vi "ni5660 Configure for Spectrum.vi"(0 "receiver info in":T1, 1 "advanced settings":T3={"window"=enum."7 Term B-Harris", "spectral lines"=-1, "RBW definition"=enum."3dB"}, 5 "center frequency (Hz)":dbl=100000000.0 format="%.2p", 7 "span (Hz)":dbl=20000000.0 format="%.2p", 9 "resolution bandwidth (Hz)":dbl=100000.0 format="%.2p", 11 "error in (no error)":errorcluster, 12 "reference level (dBm)":i32, 13 "auto attenuation":enum16{"DISABLE", "ENABLE"}(ring)=enum."ENABLE", 14 "attenuation (dB)":i32=20) -> (4 "receiver info out":T1, 8 "actual resolution bandwidth (Hz)":dbl, 10 "correction factor":T2[](array[typedef]) {"spectrum correction"."correction factors" format="%.2f"; "spectrum correction"."df" format="%.2f"; "spectrum correction"."f0" format="%.2f"}, 15 "error out":errorcluster)   [LabVIEW 2011]
doc: "This VI configures the RF Signal Analyzer hardware to acquire a frequency-domain spectrum with spectral settings you specify.<B> Center frequency</B>, <B>span</B>, and <B>resolution bandwidth</B> parameter settings define the spectrum. You can also specify window type, number of spectral lines, and resolution bandwidth (RBW) definition. \n\nThis VI configures the reference level and attenuation settings used by the RF downconverter module, and the horizontal settings and acquisition type used by the IF digitizer module. It returns a <B>correction factor</B> array. Wire this output to the <B>correction factor</B> input parameter of the ni5660 Read Averaged Power Spectrum VI or ni5660 Read FFT Spectrum VI."
uses:
  <vilib>/addons/Spectral Measurements Toolset/LVSupport/SMT niScope Utilities/smt_correction.ctl
  <vilib>/addons/Modulation/niScope/controls/mod_Modulation Settings.ctl
  <vilib>/addons/Spectral Measurements Toolset/LVSupport/SMT niScope Utilities/SMT niScope Dependent/SMT Config niScope for Spectrum(auto).vi
  <instrlib>/NITUNER/niTuner Get Cal.vi
  <instrlib>/NITUNER/niTuner Set Freq.vi
  <vilib>/Analysis/1siggen.llb/Ramp Pattern by Samples.vi
  <vilib>/addons/Spectral Measurements Toolset/LVSupport/SMT niScope Utilities/SMT Calculate Correction(Zoom FFT).vi
  <vilib>/addons/Spectral Measurements Toolset/LVSupport/SMT niScope Utilities/SMT RFSA Dependent/SMT Configure RFSA for Spectrum(auto).vi
  <vilib>/Analysis/NI_AALBase.lvlib
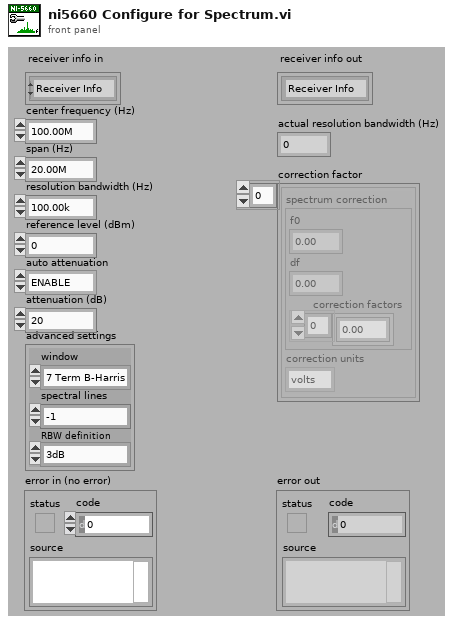
[diagram p1: front panel]
types:
  T1 = typedef "mod_Modulation Settings.ctl" = cluster{enum16{"Receiver Info"}, variant}
  T2 = typedef "smt_correction.ctl" = cluster{"spectrum correction":cluster{"f0":dbl, "df":dbl, "correction factors":dbl[]}, "correction units":enum16{"volts", "watts", "dB"}}
  T3 = cluster{"window":enum16{"None ", "Hanning", "Hamming", "Blackman-Harris", "Exact Blackman", "Blackman", "Flat Top", "4 Term B-Harris ", "7 Term B-Harris", "Low Sidelobe"}, "spectral lines":i32, "RBW definition":enum16{"3dB", "6dB", "ENBW", "bin width"}}
  T4 = cluster{"window":enum16{"None ", "Hanning", "Hamming", "Blackman-Harris", "Exact Blackman", "Blackman", "Flat Top", "4 Term B-Harris ", "7 Term B-Harris", "Low Sidelobe"}, "spectral lines":i32, "effective band specification":cluster{"fl":dbl, "fh":dbl}, "RBW definition":enum16{"3dB", "6dB", "ENBW", "bin width"}}
  T5 = cluster{"multispan?":bool, "segment size":dbl, "number of segments":i32, "frequency shifts":dbl[], "fc adjustment":dbl, "df":dbl, "start frequency (Hz)":dbl, "stop frequency (Hz)":dbl}
  T6 = enum16{"Volts", "Watts", "dBm", "dBW", "dBV", "dBmV", "dBuV"}
  T7 = enum32{"software", "RTSI 0", "RTSI 1", "RTSI 2", "RTSI 3", "RTSI 4", "RTSI 5", "RTSI 6", "no change"}
  T8 = typedef "mod_Readable Attributes Cluster.ctl" = cluster{"carrier":cluster{"frequency":dbl}, "receiver":cluster{"handles":cluster{"niTuner taskID":i32, "niScope handle":refnum<k15>}, "RFSA":cluster{"reference level":i32, "RF attenuation":i32}, "data format":enum16{"real", "complex modulated (array)", "complex modulated (interleaved)"}, "auto suppress SW IQ":enum16{"off", "on"}, "IQ sample rate":dbl, "bandwidth":dbl}}
  T9 = enum16{"None ", "Hanning", "Hamming", "Blackman-Harris", "Exact Blackman", "Blackman", "Flat Top", "4 Term B-Harris ", "7 Term B-Harris", "Low Sidelobe"}
  T10 = cluster{"f1":dbl, "f2":dbl, "array":sgl[], "type":enum16{"LUT", "polynomial"}, "units":enum16{"Volts", "Watts", "dBm", "dBW", "dBV", "dBmV", "dBuV"}, "source":string}[][]
  T11 = cluster{"Numeric":dbl, dbl, "resolution bandwidth (Hz)":dbl}
  T12 = cluster{"f1":dbl, "f2":dbl, "array":sgl[], "type":enum16{"LUT", "polynomial"}, "units":enum16{"Volts", "Watts", "dBm", "dBW", "dBV", "dBmV", "dBuV"}, "source":string}[]
  T13 = cluster{"center frequency":dbl, "span":dbl, "resolution bandwidth":dbl, "window":enum16{"None ", "Hanning", "Hamming", "Blackman-Harris", "Exact Blackman", "Blackman", "Flat Top", "4 Term B-Harris ", "7 Term B-Harris", "Low Sidelobe"}, "spectral lines":i32}
  T14 = typedef "NI_MAPro.lvlib/ma_sml_ND Zoom FFT Settings.ctl" = cluster{"zoom settings":cluster{"center frequency":dbl, "zoom":i32, "trim":dbl}, "FFT settings":cluster{"window":u16, "FFT size":i32}}
  T15 = cluster{"zoom FFT settings":T14, "frequency shift":dbl, "data format":enum16{"real", "complex modulated (array)", "complex modulated (interleaved)"}}
  T16 = enum16{"real", "complex modulated (array)", "complex modulated (interleaved)"}
  T17 = cluster{"f1":dbl, "f2":dbl, "array":sgl[], "type":enum16{"LUT", "polynomial"}, "units":enum16{"Volts", "Watts", "dBm", "dBW", "dBV", "dBmV", "dBuV"}, "source":string}
  T18 = cluster{"center frequency (Hz)":dbl, "span (Hz)":dbl, "resolution bandwidth (Hz)":dbl}
  T19 = typedef "smt_calibration.ctl" = cluster{"f1":dbl, "f2":dbl, "array":sgl[], "type":enum16{"LUT", "polynomial"}, "units":enum16{"Volts", "Watts", "dBm", "dBW", "dBV", "dBmV", "dBuV"}, "source":string}
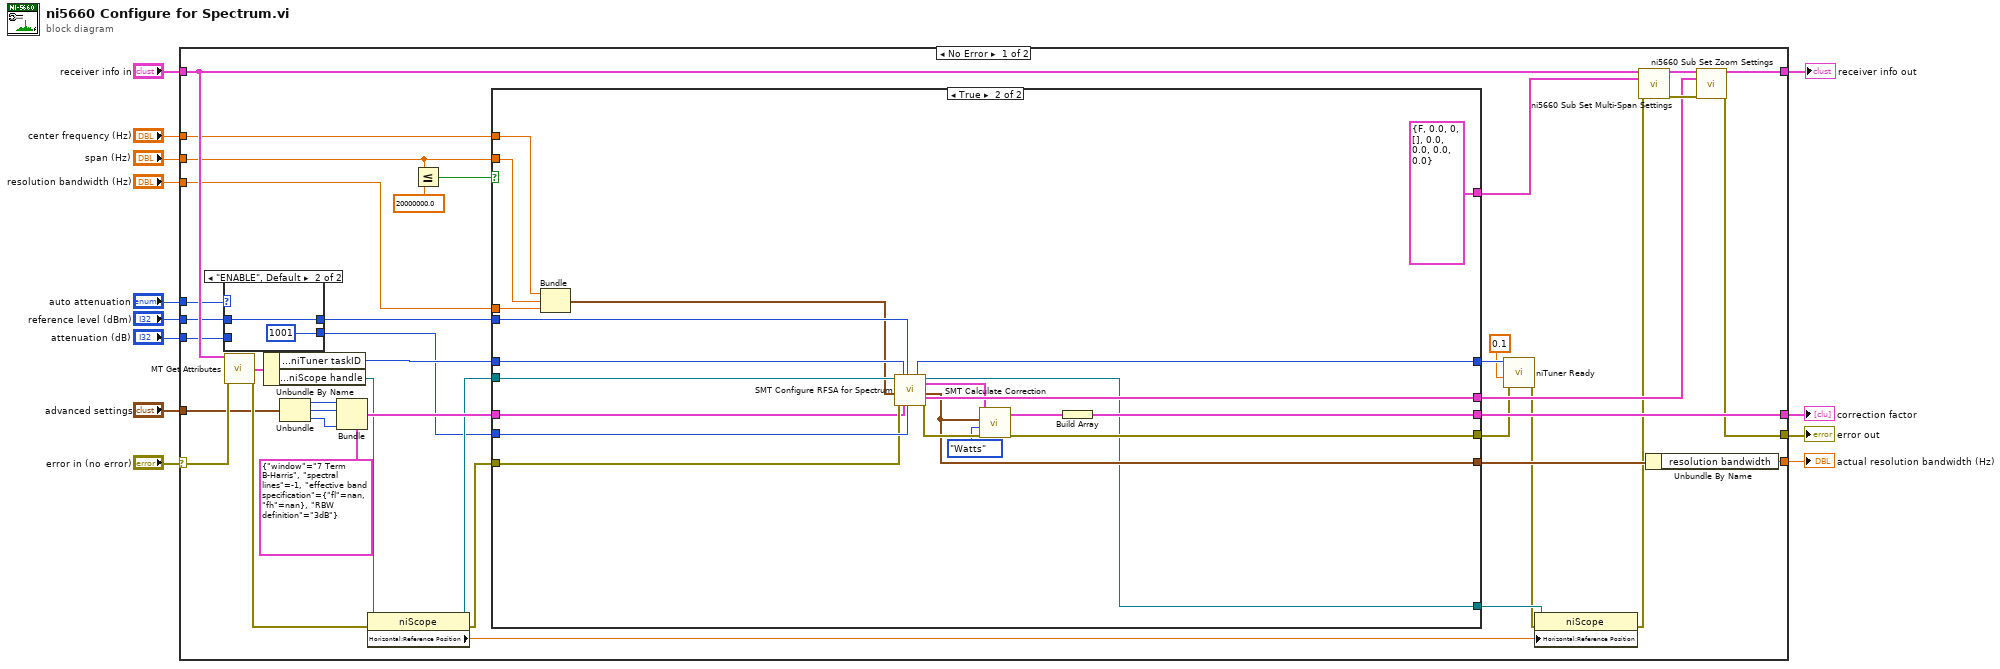
[diagram p0: block diagram]
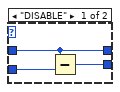
[diagram p2: hidden frame]
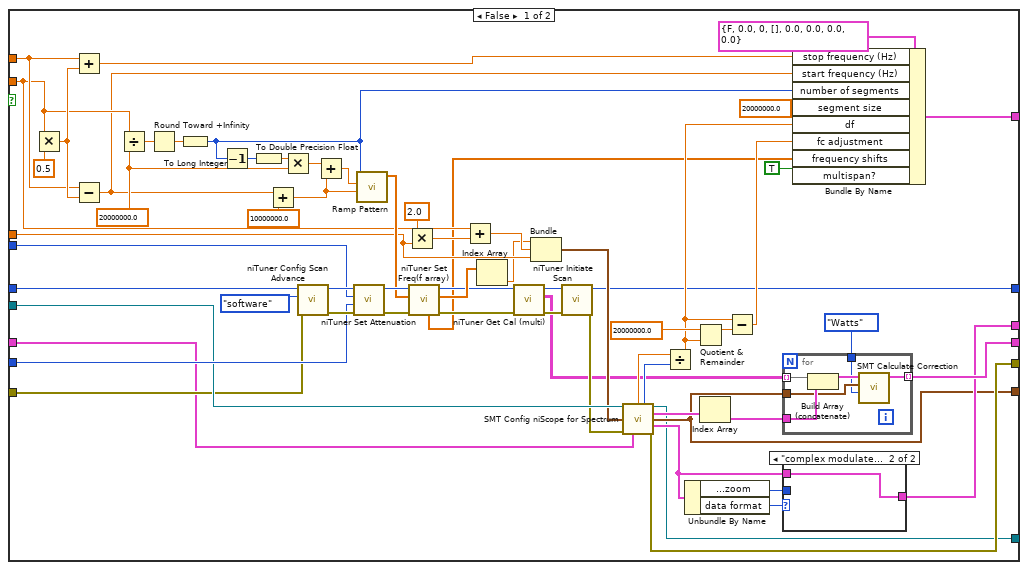
[diagram p3: hidden frame]
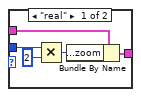
[diagram p4: hidden frame]
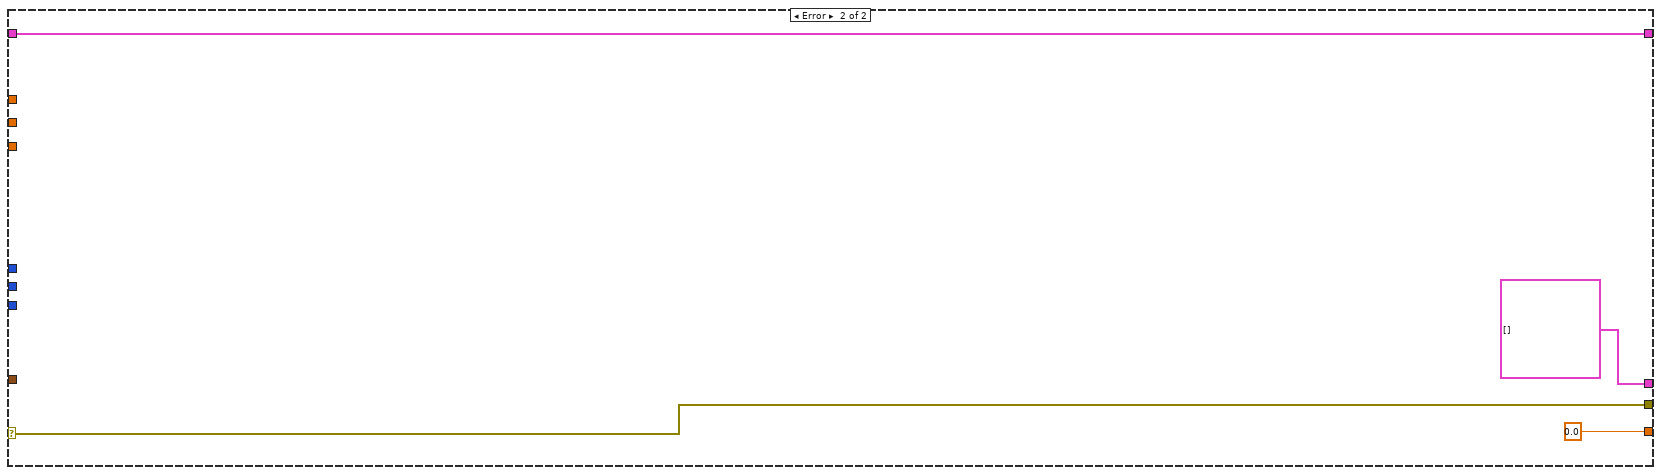
[diagram p5: hidden frame]
diagram:
  n1 = case shown="No Error" "error in (no error)" {
    selector: "error in (no error)" -> [w48 w159]
    tunnel: "reference level (dBm)" -> [w21 _]
    tunnel: [w51 T2[] []] -> w11
    tunnel: [w46 w159] -> w10
    tunnel: "receiver info in" -> [w43 w158]
    tunnel: [w45 w158] -> w8
    tunnel: [w38 0.0 ("resolution bandwidth")] -> w7
    tunnel: "advanced settings" -> [w30 _]
    tunnel: "center frequency (Hz)" -> [w25 _]
    tunnel: "span (Hz)" -> [w24 _]
    tunnel: "resolution bandwidth (Hz)" -> [w23 _]
    tunnel: "attenuation (dB)" -> [w20 _]
    tunnel: "auto attenuation" -> [w22 _]
    frame No Error {
      n2 = case shown="\"ENABLE\", Default" w22 {
        tunnel: w21 -> [w55 w58]
        tunnel: w20 -> [w56 _]
        tunnel: [w55 w58] -> w19
        tunnel: [w54 1001] -> w18
        frame "DISABLE" {
          n3 = Subtract(x=w55, y=w56) -> (x-y=w54:i32)
        }
        frame "ENABLE", Default {
        }
      }
      n4 = call <vilib>:"MT Get Attributes.vi"("receiver info in"=w43, "error in (no error)"=w48) -> ("attributes"=w49:T8, "error out"=w35:errorcluster)  [unwired: 11 in, 1 out]
      n5 = Unbundle By Name(w49) -> ("receiver.handles.niTuner taskID"=w47:i32, "receiver.handles.niScope handle"=w37:refnum<k15>)
      n6 = Unbundle(w30) -> ("window"=w28:T9, "spectral lines"=w27:i32, "RBW definition"=w26:enum16{"3dB", "6dB", "ENBW", "bin width"})
      n7 = Bundle(cluster=T4 {"window"=enum."7 Term B-Harris", "spectral lines"=-1, "effective band specification"={"fl"=nan, "fh"=nan}, "RBW definition"=enum."3dB"} ("advanced settings"), "window"=w28, "spectral lines"=w27, "RBW definition"=w26) -> (w50:T4)  [unwired: 1 in]
      n8 = property class="niScope"(reference=w37, error in=w35) -> (reference out=w36:refnum<k15>, error out=w34:errorcluster, "Horizontal:Reference Position"=w33:dbl)
      n9 = Less Or Equal?(x=w24, y=20000000.0) -> (x <= y?=w52:bool)
      n10 = case shown="True" w52 {
        tunnel: w47 -> [w121 w154]
        tunnel: w36 -> [w95 w155]
        tunnel: w19 -> [w119 w153]
        tunnel: w18 -> [w118 w152]
        tunnel: w34 -> [w77 w151]
        tunnel: [w79 w150] -> w40
        tunnel: [w80 w141] -> w15
        tunnel: w24 -> [w74 w138]
        tunnel: w25 -> [w100 w137]
        tunnel: w23 -> [w98 w139]
        tunnel: [w81 w145] -> w51
        tunnel: [w78 w144] -> w39
        tunnel: w50 -> [w76 w143]
        tunnel: [w66 T5 {"multispan?"=FALSE, "segment size"=0.0, "number of segments"=0, "frequency shifts"=[], "fc adjustment"=0.0, "df"=0.0, "start frequency (Hz)"=0.0, "stop frequency (Hz)"=0.0} ("multispan settings")] -> w44
        tunnel: [w64 w140] -> w32
        tunnel: [w59 w135] -> w17
        frame False {
          w105 = 20000000.0 ("y")
          n11 = Multiply(x=w74, y=0.5 ("x")) -> (x*y=w103:dbl)
          n12 = Add(x=w100, y=w103) -> (x+y=w75:dbl)
          n13 = Subtract(x=w100, y=w103) -> (x-y=w73:dbl)
          n14 = Divide(x=w74, y=w105) -> (x/y=w109:dbl)
          n15 = Round Toward +Infinity(x=w109) -> (ceil(x): smallest int >= x=w108:dbl)
          n16 = To Long Integer(number=w108) -> (32bit integer=w72:i32)
          n17 = Decrement(x=w72) -> (x-1=w113:i32)
          n18 = To Double Precision Float(number=w113) -> (double precision float=w112:dbl)
          n19 = Add(x=w73, y=10000000.0 ("x")) -> (x+y=w106:dbl)
          n20 = Multiply(x=w112, y=w105) -> (x*y=w111:dbl)
          n21 = call <instrlib>:"niTuner Config Scan Advance.vi"("error in"=w77, "advance trigger"=T7."software" ("Advance Trigger"), "taskID in"=w121) -> ("error out"=w122:errorcluster, "taskID out"=w120:i32)  [unwired: 7 in]
          n22 = Add(x=w111, y=w106) -> (x+y=w110:dbl)
          n23 = call <instrlib>:"niTuner Set Attenuation.vi"("error in"=w122, "mixer level (dBm)"=w118, "ref level (dBm)"=w119, "taskID in"=w120) -> ("error out"=w115:errorcluster, "taskID out"=w116:i32)  [unwired: 4 in, 2 out]
          n24 = call-poly <vilib>:"Ramp Pattern.vi"("start"=w106, "end"=w110, "samples"=w72) -> ("Ramp Pattern"=w114:dbl[])  [unwired: 7 in, 1 out]
          n25 = Multiply(x=2.0, y=w98) -> (x*y=w102:dbl)
          n26 = call-poly <instrlib>:"niTuner Set Freq(f array).vi"("error in"=w115, "desired RF frequencies"=w114, "taskID in"=w116) -> ("error out"=w83:errorcluster, "actual IF frequencies"=w99:dbl[], "taskID out"=w84:i32, "frequency shifts"=w68:dbl[])  [unwired: 4 in, 1 out]
          n27 = Add(x=w74, y=w102) -> (x+y=w97:dbl)
          n28 = Index Array(array=w99) -> (element=w96:dbl)  [unwired: 1 in]
          n29 = call-poly <instrlib>:"niTuner Get Cal (multi).vi"("error in"=w83, "taskID in"=w84) -> ("error out"=w63:errorcluster, "calibrations"=w60:T10, "taskID out"=w62:i32)  [unwired: 7 in]
          n30 = Bundle("Numeric"=w96, w97, "resolution bandwidth (Hz)"=w98) -> (w94:T11)  [unwired: 1 in]
          n31 = call <instrlib>:"niTuner Initiate Scan.vi"("error in"=w63, "taskID in"=w62) -> ("error out"=w61:errorcluster, "taskID out"=w59:i32)  [unwired: 8 in]
          n32 = call-poly <vilib>:"SMT Config niScope for Spectrum.vi"("instrument handle"=w95, "spectrum settings"=w94, "error in (no error)"=w61, "advanced settings"=w76) -> ("actual sample rate"=w93:dbl, "acquisition size"=w92:i32, "instrument handle out"=w64:refnum<k15>, "calibration array"=w85:T12, "actual spectrum settings"=w78:T13, "SMT zoom settings"=w87:T15, "error out"=w80:errorcluster)  [unwired: 5 in]
          n33 = Divide(x=w93, y=w92) -> (x/y=w70:dbl)
          n34 = Unbundle By Name(w87) -> ("zoom FFT settings.zoom settings.zoom"=w88:i32, "data format"=w89:T16)
          n35 = Quotient & Remainder(x=20000000.0 ("y"), y=w70) -> (x-y*floor(x/y)=w91:dbl)  [unwired: 1 out]
          n36 = Index Array(array=w85) -> (element=w86:T17)  [unwired: 1 in]
          n37 = Subtract(x=w70, y=w91) -> (x-y=w69:dbl)
          n38 = for {
            tunnel: w86 -> [w128]
            tunnel: [w127] -> w81 mode=indexing
            tunnel: w78 -> [w126]
            tunnel: w60 -> [w124] mode=indexing
            tunnel: T6."Watts" ("units") -> [w123]
            n39 = Build Array (concatenate)(w124, w128) -> (w125:T12)
            n40 = call-poly <vilib>:"SMT Calculate Correction.vi"("units"=w123, "actual spectrum settings"=w126, "calibration array"=w125) -> ("correction"=w127:T2)  [unwired: 7 in, 1 out]
          }
          n41 = case shown="\"complex modulated (array)\", Default" w89 {
            tunnel: w88 -> [w133 _]
            tunnel: [w130 w134] -> w79
            tunnel: w87 -> [w129 w134]
            frame "real" {
              n42 = Multiply(x=w133, y=2 ("x")) -> (x*y=w131:i32)
              n43 = Bundle By Name(cluster=w129, "zoom FFT settings.zoom settings.zoom"=w131) -> (w130:T15)
            }
            frame "complex modulated (array)", Default {
            }
          }
          n44 = Bundle By Name(cluster=T5 {"multispan?"=FALSE, "segment size"=0.0, "number of segments"=0, "frequency shifts"=[], "fc adjustment"=0.0, "df"=0.0, "start frequency (Hz)"=0.0, "stop frequency (Hz)"=0.0} ("multispan settings"), "stop frequency (Hz)"=w75, "start frequency (Hz)"=w73, "number of segments"=w72, "segment size"=20000000.0 ("y"), "df"=w70, "fc adjustment"=w69, "frequency shifts"=w68, "multispan?"=TRUE) -> (w66:T5)
        }
        frame True {
          n45 = Bundle("center frequency (Hz)"=w137, "span (Hz)"=w138, "resolution bandwidth (Hz)"=w139) -> (w136:T18)  [unwired: 1 in]
          n46 = call-poly <vilib>:"SMT Configure RFSA for Spectrum.vi"("instrument handle"=w155, "spectrum settings"=w136, "error in (no error)"=w151, "tuner taskID"=w154, "advanced settings"=w143, "ref level (dBm)"=w153, "mixer level (dBm)"=w152) -> ("tuner taskID out"=w135:i32, "instrument handle out"=w140:refnum<k15>, "calibration array"=w149:T19[], "actual spectrum settings"=w144:T13, "SMT zoom settings"=w150:T15, "error out"=w148:errorcluster)  [unwired: 5 in, 2 out]
          n47 = call-poly <vilib>:"SMT Calculate Correction.vi"("error in (no error)"=w148, "units"=T6."Watts", "actual spectrum settings"=w144, "calibration array"=w149) -> ("error out"=w141:errorcluster, "correction"=w146:T2)  [unwired: 6 in]
          n48 = Build Array(w146) -> (w145:T2[])
        }
      }
      n49 = call <instrlib>:"niTuner Ready.vi"("error in"=w15, "timeout"=0.1, "taskID in"=w17) -> ("error out"=w16:errorcluster)  [unwired: 6 in, 2 out]
      n50 = property class="niScope"(reference=w32, error in=w16, "Horizontal:Reference Position"=w33) -> (error out=w31:errorcluster)  [unwired: 1 out]
      n51 = call <instrlib>:"ni5660 Sub Set Multi-Span Settings.vi"("receiver info in"=w43, "multispan settings"=w44, "error in (no error)"=w31) -> ("receiver info out"=w42:T1, "error out"=w41:errorcluster)  [unwired: 11 in]
      n52 = Unbundle By Name(w39) -> ("resolution bandwidth"=w38:dbl)
      n53 = call <instrlib>:"ni5660 Sub Set Zoom Settings.vi"("receiver info in"=w42, "zoom settings"=w40, "error in (no error)"=w41) -> ("receiver info out"=w45:T1, "error out"=w46:errorcluster)  [unwired: 11 in]
    }
    frame Error {
    }
  }
  "error out" <- w10
  "correction factor" <- w11
  "receiver info out" <- w8
  "actual resolution bandwidth (Hz)" <- w7
